vi "Measure Voltage (Average).vi"(8 "error in (no error)":errorcluster, 9 "Sample Count (1)":i32=1, 10 "Channel List (101:110)":string="107", 11 "DMM":refnum<visa-resource-name>="COM1") -> (0 "error out":errorcluster, 1 "Voltage":dbl format="%0.8f", 2 "Voltage Data":dbl[](array[numeric]))   [LabVIEW 2015]
uses:
  <instrlib>/Keithley 27XX/Public/Data/Read Multiple Direct.vi
  <vilib>/measure/madcrms.llb/Basic Averaged DC-RMS for 1 Chan.vi
  <instrlib>/Keithley 27XX/Keithley 27XX.lvlib
  <vilib>/measure/NI_MAPro.lvlib
panel:
  in  "Serial Configuration":T1={"Baud Rate (19200)"=19200, "Flow Control (1: XON/XOFF)"=1, "Termination Char (0:CR)"=0} {"Termination Char (0:CR)" items=["CR", "LF"]; "Flow Control (1: XON/XOFF)" items=["None", "XON/XOFF", "RTS/CTS (2701 Only)", "XON/XOFF & RTS/CTS (2701 Only)"]; "Baud Rate (19200)" items=["300"=300, "600"=600, "1200"=1200, "2400"=2400, "4800"=4800, "9600"=9600, "19.2k"=19200, "38.4k (2701 Only)"=38400, "57.6k (2701 Only)"=57600, "115.2k (2701 Only)"=115200]}
  in  "Timeout (5000 milliseconds)":u32=5000
  in  "Function (0: DC Voltage)":u16(ring) items=["DC Voltage", "AC Voltage", "DC Current", "AC Current", "Resistance", "Four-Wire Resistance", "Temperature (C)", "Frequency", "Period", "Continuity"]
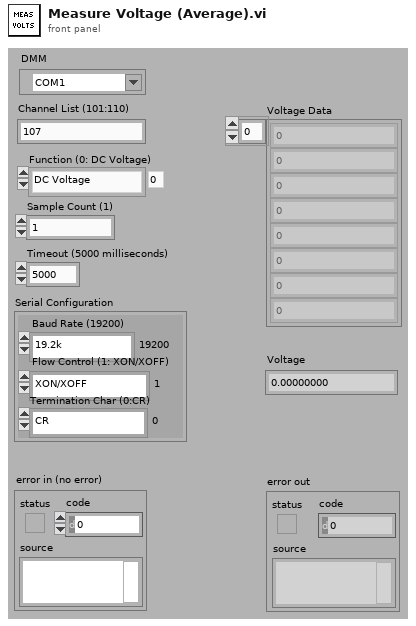
[diagram p1: front panel]
types:
  T1 = cluster{"Baud Rate (19200)":u32, "Flow Control (1: XON/XOFF)":u16, "Termination Char (0:CR)":u16}
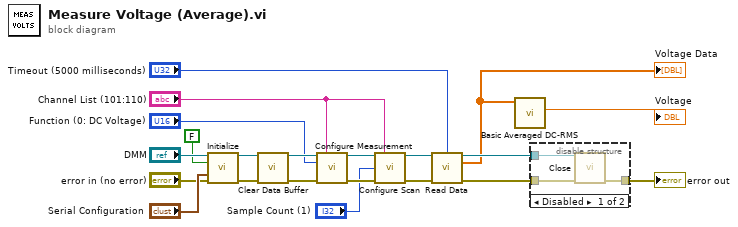
[diagram p0: block diagram]
diagram:
  n1 = call <instrlib>:"Initialize.vi"("VISA resource name"="DMM", "ID Query? (T: Yes)"=FALSE, "Serial Configuration"="Serial Configuration", "error in (no error)"="error in (no error)") -> ("VISA resource name out"=w14:refnum<visa-resource-name>, "error out"=w15:errorcluster)  [unwired: 10 in]
  n2 = call <instrlib>:"Clear Data Buffer.vi"("VISA resource name"=w14, "error in (no error)"=w15) -> ("VISA resource name out"=w17:refnum<visa-resource-name>, "error out"=w16:errorcluster)  [unwired: 12 in]
  n3 = call <instrlib>:"Configure Measurement.vi"("VISA resource name"=w17, "Scan List (Empty)"="Channel List (101:110)", "Function (0: DC Voltage)"="Function (0: DC Voltage)", "error in (no error)"=w16) -> ("VISA resource name out"=w21:refnum<visa-resource-name>, "error out"=w18:errorcluster)  [unwired: 10 in]
  n4 = call <instrlib>:"Configure Scan.vi"("VISA resource name"=w21, "Channel List (101:110)"="Channel List (101:110)", "Sample Count (100)"="Sample Count (1)", "error in (no error)"=w18) -> ("VISA resource name out"=w11:refnum<visa-resource-name>, "error out"=w12:errorcluster)  [unwired: 10 in]
  n5 = call-poly <instrlib>:"Read Data.vi"("VISA resource name"=w11, "Timeout (30000 milliseconds)"="Timeout (5000 milliseconds)", "error in (no error)"=w12) -> ("VISA resource name out"=w20:refnum<visa-resource-name>, "Measurement Data"=w2:dbl[], "error out"=w19:errorcluster)  [unwired: 7 in, 3 out]
  "Voltage Data" <- w2
  n6 = call-poly <vilib>:"Basic Averaged DC-RMS.vi"("signal in"=w2) -> ("RMS value"=→"Voltage":dbl)  [unwired: 7 in, 3 out]
  n7 = disable-structure shown="Disabled" {
    disable-tunnel: w20 -> [w24 _]
    disable-tunnel: w19 -> [w23 w25]
    disable-tunnel: [w22 w25] -> w6
    frame Disabled {
      n8 = call <instrlib>:"Close.vi"("VISA resource name"=w24, "error in (no error)"=w23) -> ("error out"=w22:errorcluster)  [unwired: 13 in]
    }
    frame Enabled {
    }
  }
  "error out" <- w6
